vi "CSM - Start File Logger.vi"(4 "Filter Rules":refnum<class "LogFilter.lvclass">, 5 "Timestamp Format":string="%<%Y/%m/%d %H:%M:%S%3u>T", 6 "Enable? (T)":bool=TRUE, 7 "Log Limit":T1={"file size (in bytes)"=10000000, "file num"=2} {"file size (in bytes)" format="%.0p"}, 8 "Error In":errorcluster caption="error in (no error)", 9 "Watchdog? (T)":bool=TRUE, 10 "Exit When All Module Exist? (F)":bool, 11 "Log File Path":path) -> (0 "error out":errorcluster, 2 "Log File":path, 3 "Watchdog Queue":refnum<queue>)   [LabVIEW 2017, in "CSM File Logger.lvlib"]
doc: "Starts the CSM Global Log file recording background thread, which is used to save all execution records in the application to a specified text file.\n\n> [!NOTE] <b>CSM File Logger Implementation Principle</b>\n>\n> The CSM File Logger retrieves all execution records in the application via the CSM Global Log API and saves them to a specified text file for later analysis and error localization. The file format is a text file with the suffix `.csmlog`, which can be opened using text editing query tools such as Notepad.\n\n> [!NOTE] <b>Log File Limits</b>\n>\n> To prevent log files from becoming too large due to long-running software, limits are set on log file size and the number of files:\n> - <b>File Size</b>: The maximum size of a single file in bytes. The default is 10 MB.\n> - <b>File Num</b>: The maximum number of LOG files. The default is 2.\n>\n> When the log file size exceeds the <b>File Size</b> limit, a new file record is created. When the number of log files exceeds the <b>File Num</b> limit, the oldest file record is deleted.\n\n\n> [!NOTE] <b>Global Log Filter Rules</b>\n>\n> Global log filter rules allow a category of logs to be filtered out so they do not appear in the global log.\n>\n> The following are the three types of log filter rules:\n> - <b>Global Rules</b>: Apply to all modules meeting the conditions. You can configure the following settings:\n> - <b>Module Name</b>: All names of the module will be filtered.\n> - <b>Log Type</b>: Such as state, message, broadcast, module Initialization, and so on.\n> - <b>State Name</b>: Any module with the state name will be filtered.\n> - <b>State Type</b>: Type of state, such as internal state, external message, and so on.\n> - <b>Broadcast</b>: Broadcasts with the specified broadcast name will be filtered. Applies to Status Broadcast and Interrupt Broadcast logs.\n> - <b>User Log</b>: User logs with the specified user log name will be filtered.\n> - <b>Module Rules</b>: Apply to specific modules. You can configure the following settings:\n> - <b>Module Log Type</b>: Modules with the specified log types of the module are filtered.\n> - <b>State Name</b>: Modules with the specified state name are filtered.\n> - <b>State Type</b>: Modules with the specified state type are filtered.\n> - <b>Broadcast</b>: Modules with the specified broadcast name are filtered.\n> - <b>User Log</b>: Modules with the specified user log name are filtered.\n> - <b>Periodic Filter Rules</b>: This rule is currently only effective at the registration point because it is difficult to count numbers at the publication location.\n> - Whether to enable periodic filtering.\n> - <b>Threshold (#/s)</b>: Periodic filtering threshold.\n> - <b>CheckPeriod (s)</b>: Check window time.\n\n\n<b>Reference Example</b>: `Addons - Logger\\CSM Application Running Log Example.vi`.\n\n-- <b>Controls</b> --\n- <b>Log File Path</b>: Log file path.\n- <b>Timestamp format</b>: Time format. The default is `%<%Y/%m/%d %H:%M:%S%3u>T`.\n- <b>Log Limit</b>: Log file size limit. <b>File Size</b> is the maximum size of a single file in bytes. The default is 10 MB. <b>File Num</b> is the maximum number of LOG files. The default is 2.\n- <b>Filter Rules</b>: Filter rules, configured via the CSM - Convert Filter Rules VI.\n- <b>Enable? (T)</b>: Whether to enable the file recording function. The default is TRUE, which specifies to enable the file recording function. When <b>Enable?</b> is FALSE, the file recording function is disabled.\n- <b>WatchDog? (T)</b>: Whether to enable the WatchDog function. The default is TRUE. When the calling VI exits, the allocated WatchDog resource is automatically released, triggering the recording thread to exit automatically; manually releasing the WatchDog resource will also trigger the recording thread to exit.\n- <b>Exit When All Module Exist? (F)</b>: Automatically exit recording after all CSM modules have exited. The default is FALSE. If TRUE, and the main program is not a CSM, the recording thread will also automatically exit when all running CSM modules exit.\n\n-- <b>Indicators</b> --\n- <b>Log File</b>: CSM LOG file path.\n- <b>Watchdog Queue</b>: WatchDog resource handle."
uses:
  CSM File Logger.lvlib
  CSM File Logger Limit.ctl
  _Support/GlobalEvent/LogFilter/LogFilter.lvclass
  _Shared/CSM Shared.lvlib
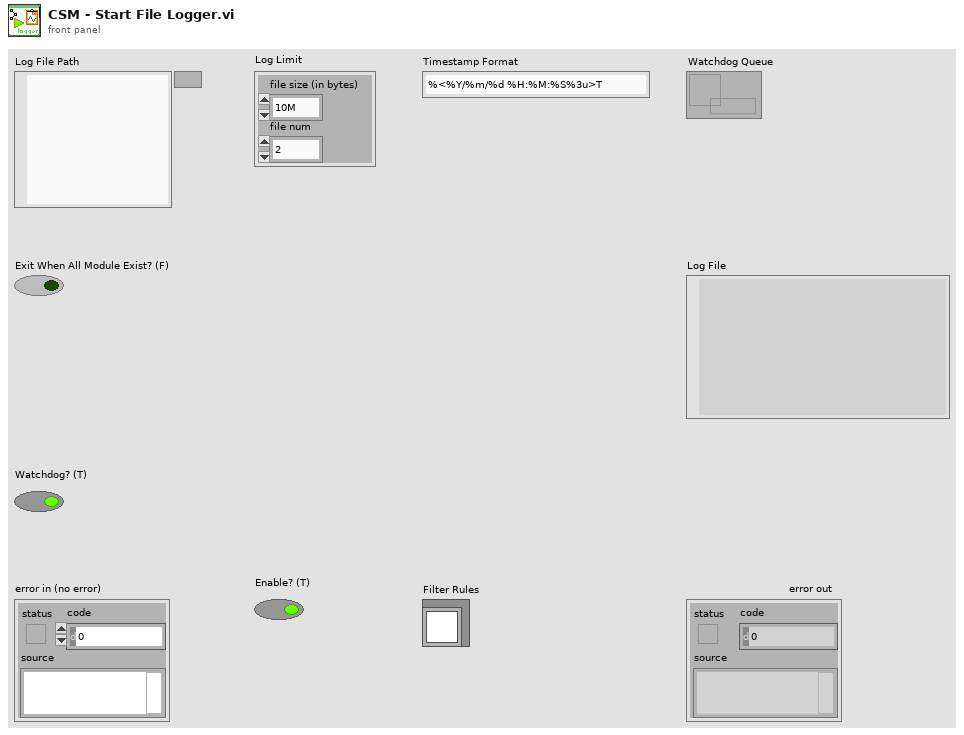
[diagram p1: front panel]
types:
  T1 = typedef "CSM File Logger.lvlib/CSM File Logger Limit.ctl" = cluster{"file size (in bytes)":i64, "file num":i32}
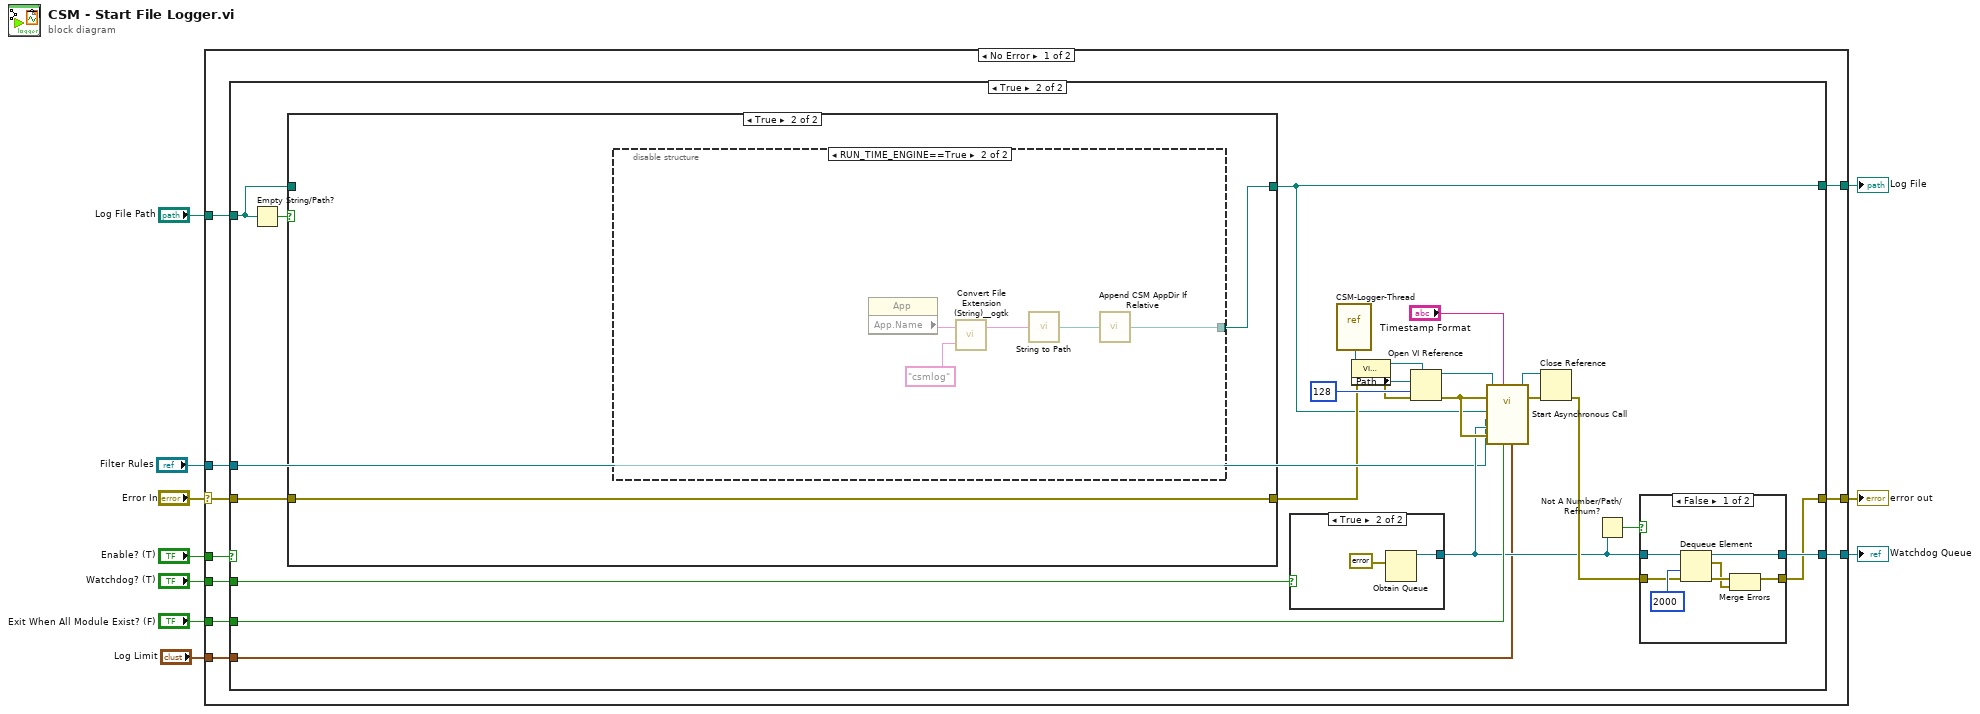
[diagram p0: block diagram]
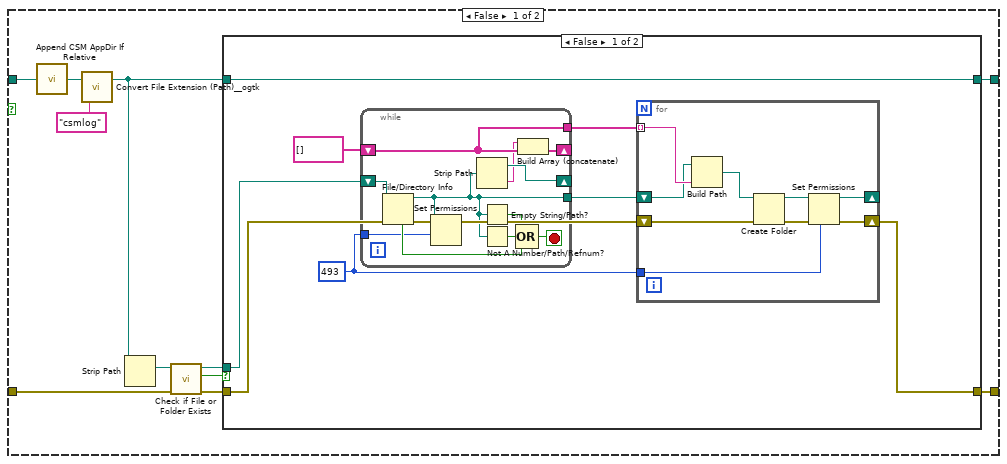
[diagram p3: hidden frame]
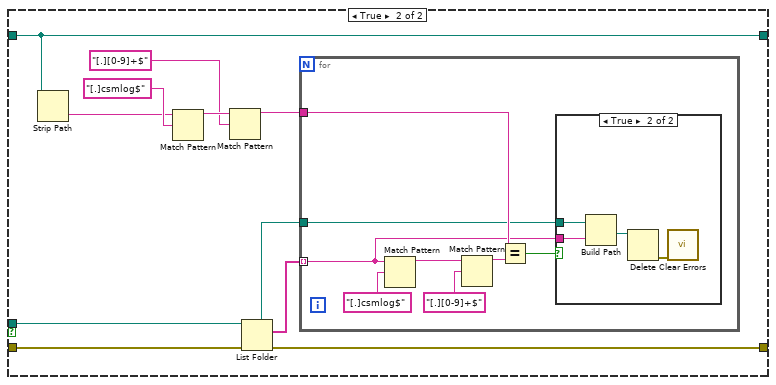
[diagram p4: hidden frame]
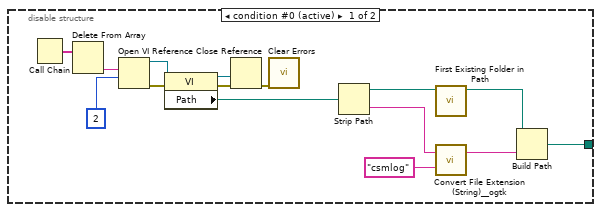
[diagram p6: hidden frame]
diagram:
  n1 = case shown="No Error" "Error In" {
    selector: "Error In" -> [w20 w141]
    tunnel: "Log File Path" -> [w18 _]
    tunnel: [w19 w141] -> w8
    tunnel: "Enable? (T)" -> [w17 _]
    tunnel: "Watchdog? (T)" -> [w16 _]
    tunnel: [w15 _] -> w2
    tunnel: "Exit When All Module Exist? (F)" -> [w14 _]
    tunnel: [w13 _] -> w4
    tunnel: "Log Limit" -> [w12 _]
    tunnel: "Filter Rules" -> [w11 _]
    frame No Error {
      n2 = case shown="True" w17 {
        tunnel: w20 -> [w21 w25]
        tunnel: [w21 w32] -> w19
        tunnel: w18 -> [_ w23]
        tunnel: w16 -> [_ w36]
        tunnel: [_ w34] -> w15
        tunnel: w14 -> [_ w35]
        tunnel: [_ w22] -> w13
        tunnel: w12 -> [_ w29]
        tunnel: w11 -> [_ w27]
        frame False {
        }
        frame True {
          n3 = Empty String/Path?(string/path=w23) -> (empty?=w26:bool)
          n4 = case shown="True" w26 {
            tunnel: w25 -> [w52 w109]
            tunnel: [w55 w109] -> w24
            tunnel: w23 -> [w54 _]
            tunnel: [w47 w108] -> w22
            frame False {
              n5 = call "Append CSM AppDir If Relative.vi"("Relative Path (.)"=w54) -> ("Application Directory (+ Relative)"=w48:path)  [unwired: 4 in]
              n6 = call "Convert File Extension (Path)__ogtk.vi"("New Ending (None)"="csmlog" ("new ending (none)"), "File Name"=w48) -> ("New Filename"=w46:path)  [unwired: 1 out]
              n7 = Strip Path(path=w46) -> (stripped path=w56:path)  [unwired: 1 out]
              n8 = call <vilib>:"Check if File or Folder Exists.vi"("error in (no error)"=w52, "path"=w56) -> ("error out"=w51:errorcluster, "file or folder exists?"=w50:bool, "dup path"=w53:path)  [unwired: 7 in]
              n9 = case shown="False" w50 {
                tunnel: [w64 w94] -> w55
                tunnel: w53 -> [w63 w93]
                tunnel: w51 -> [w62 w95]
                tunnel: [w61 w86] -> w47
                tunnel: w46 -> [w61 w86]
                frame False {
                  w60 = i16 493 ("permissions (0755)")
                  n10 = while {
                    shift-right: [w68] -> _
                    shift-left: w63 -> [w75]
                    shift-right: [w74] -> _
                    shift-left: string[] [] -> [w73]
                    tunnel: [w73] -> w58
                    tunnel: [w66] -> w59
                    tunnel: w60 -> [w65]
                    stop <- w72 stop-if-true
                    n11 = File/Directory Info(path=w75) -> (path out=w66:path, directory=w69:bool)  [unwired: 1 in, 5 out]
                    n12 = Set Permissions(7:w65, 11:w66) -> ()  [unwired: 3 in, 2 out]
                    n13 = Strip Path(path=w66) -> (stripped path=w68:path, name=w67:string)
                    n14 = Empty String/Path?(string/path=w66) -> (empty?=w71:bool)
                    n15 = Not A Number/Path/Refnum?(number/path/refnum=w66) -> (NaN/Path/Refnum?=w70:bool)
                    n16 = Compound Arithmetic op=OR(w71, w70, w69) -> (w72:bool)
                    n17 = Build Array (concatenate)(w67, w73) -> (w74:string[])
                  }
                  n18 = for {
                    tunnel: w58 -> [w84] mode=indexing
                    shift-right: [w78] -> _
                    shift-left: w59 -> [w83]
                    shift-right: [w82] -> w64
                    shift-left: w62 -> [w81]
                    tunnel: w60 -> [w79]
                    n19 = Build Path(base path=w83, name or relative path=w84) -> (appended path=w80:path)
                    n20 = Create Folder(path (use dialog)=w80, error in=w81) -> (created path=w77:path, error out=w76:errorcluster)  [unwired: 1 in, 1 out]
                    n21 = Set Permissions(7:w79, 8:w76, 11:w77) -> (0:w82:errorcluster, 3:w78:path)  [unwired: 2 in]
                  }
                }
                frame True {
                  n22 = Strip Path(path=w86) -> (name=w88:string)  [unwired: 1 out]
                  n23 = Match Pattern(string=w88, regular expression="[.]csmlog$") -> (before substring=w91:string)  [unwired: 1 in, 3 out]
                  n24 = Match Pattern(string=w91, regular expression="[.][0-9]+$") -> (before substring=w85:string)  [unwired: 1 in, 3 out]
                  n25 = List Folder(path=w93, error in=w95) -> (path out=w87:path, filenames=w92:string[], error out=w94:errorcluster)  [unwired: 2 in, 1 out]
                  n26 = for {
                    tunnel: w92 -> [w96] mode=indexing
                    tunnel: w85 -> [w99]
                    tunnel: w87 -> [w97]
                    n27 = Match Pattern(string=w96, regular expression="[.]csmlog$") -> (before substring=w103:string)  [unwired: 1 in, 3 out]
                    n28 = Match Pattern(string=w103, regular expression="[.][0-9]+$") -> (before substring=w100:string)  [unwired: 1 in, 3 out]
                    n29 = Equal?(x=w99, y=w100) -> (x = y?=w98:bool)
                    n30 = case shown="True" w98 {
                      tunnel: w97 -> [_ w106]
                      tunnel: w96 -> [_ w105]
                      frame False {
                      }
                      frame True {
                        n31 = Build Path(base path=w106, name or relative path=w105) -> (appended path=w107:path)
                        n32 = Delete(path (use dialog)=w107) -> (error out=w104:errorcluster)  [unwired: 4 in, 2 out]
                        n33 = call <vilib>:"Clear Errors.vi"("error in (no error)"=w104) -> ()  [unwired: 5 in, 2 out]
                      }
                    }
                  }
                }
              }
            }
            frame True {
              n34 = disable-structure shown="RUN_TIME_ENGINE==True" {
                disable-tunnel: [w115 w126] -> w108
                frame condition #0 (active) {
                  n35 = Call Chain() -> (call chain=w123:string[])
                  n36 = Delete From Array(array=w123) -> (deleted portion=w122:string)  [unwired: 2 in, 1 out]
                  n37 = Open VI Reference(vi path=w122, options=2) -> (vi reference=w119:refnum<vi>, error out=w120:errorcluster)  [unwired: 4 in]
                  n38 = property class="VI"(reference=w119, error in=w120) -> (reference out=w117:refnum<vi>, error out=w118:errorcluster, "Path"=w124:path)
                  n39 = Close Reference(reference=w117, error in (no error)=w118) -> (error out=w116:errorcluster)
                  n40 = call <vilib>:"Clear Errors.vi"("error in (no error)"=w116) -> ()  [unwired: 5 in, 2 out]
                  n41 = Strip Path(path=w124) -> (stripped path=w114:path, name=w112:string)
                  n42 = call "First Existing Folder in Path.vi"("Stripped Path In"=w114) -> ("Stripped Path Out"=w111:path)  [unwired: 10 in]
                  n43 = call "Convert File Extension (String)__ogtk.vi"("New Ending (None)"="csmlog" ("new ending (none)"), "File Name"=w112) -> ("New Filename"=w110:string)  [unwired: 1 out]
                  n44 = Build Path(base path=w111, name or relative path=w110) -> (appended path=w115:path)
                }
                frame condition #1 {
                  n45 = property class="App"() -> ("App.Name"=w128:string)  [unwired: 2 in, 2 out]
                  n46 = call "Convert File Extension (String)__ogtk.vi"("New Ending (None)"="csmlog" ("new ending (none)"), "File Name"=w128) -> ("New Filename"=w127:string)  [unwired: 1 out]
                  n47 = call "String to Path.vi"("String"=w127) -> ("Path"=w125:path)
                  n48 = call "Append CSM AppDir If Relative.vi"("Relative Path (.)"=w125) -> ("Application Directory (+ Relative)"=w126:path)  [unwired: 4 in]
                }
              }
            }
          }
          n49 = case shown="True" w36 {
            tunnel: [_ w131] -> w31
            frame False {
            }
            frame True {
              n50 = Obtain Queue(element data type=errorcluster {"status"=FALSE, "code"=0, "source"=""} ("error in (no error)")) -> (queue out=w131:refnum<queue>)  [unwired: 4 in, 2 out]
            }
          }
          n51 = vi-ref "CSM-Logger-Thread.vi"() -> (w39:refnum<vi>)
          n52 = property class="VI (strict)"(reference=w39, error in=w24) -> (reference out=w43:refnum<vi>, error out=w41:errorcluster, "Path"=w40:path)
          n53 = Open VI Reference(type specifier VI Refnum (for type only)=w43, vi path=w40, options=128, error in (no error)=w41) -> (vi reference=w38:refnum<vi>, error out=w44:errorcluster)  [unwired: 2 in]
          n54 = call-by-ref "Start Asynchronous Call"(reference=w38, error in=w44, "log limit"=w29, "Exit When All Module Exist?(F)"=w35, "format string"="Timestamp Format", 8:"error in (no error)"=w44, "WatchDogQ"=w31, "GlobalLogFilter.lvclass"=w27, "file path (use dialog)"=w22) -> (reference out=w37:refnum<vi>, error out=w42:errorcluster)  [unwired: 4 in, 1 out]
          n55 = Close Reference(reference=w37, error in (no error)=w42) -> (error out=w33:errorcluster)
          n56 = Not A Number/Path/Refnum?(number/path/refnum=w31) -> (NaN/Path/Refnum?=w30:bool)
          n57 = case shown="False" w30 {
            tunnel: [w138 w140] -> w34
            tunnel: w33 -> [w136 w139]
            tunnel: [w133 w139] -> w32
            tunnel: w31 -> [w134 w140]
            frame False {
              n58 = Dequeue Element(queue=w134, timeout in ms (-1)=2000, error in (no error)=w136) -> (queue out=w138:refnum<queue>, element=w132:errorcluster, error out=w135:errorcluster)  [unwired: 1 out]
              n59 = Merge Errors(w135, w132) -> (w133:errorcluster)
            }
            frame True {
            }
          }
        }
      }
    }
    frame Error {
    }
  }
  "error out" <- w8
  "Watchdog Queue" <- w2
  "Log File" <- w4
